vi "NewSolutionFitness.vi"(8 "error in (no error)":errorcluster, 10 "OSSP_Problem.lvclass":refnum<class "OSSP_Problem.lvclass">, 11 "GA in":refnum<class "GA.lvclass">) -> (0 "error out":errorcluster, 2 "OSSP_Problem out":refnum<class "OSSP_Problem.lvclass">, 3 "GA out":refnum<class "GA.lvclass">)   [LabVIEW 2013, in "GA.lvclass"]
uses:
  GA.lvclass
  OSSP_Problem.lvclass
  GA.lvclass/GA.ctl
  OSSP_Problem.lvclass/OSSP_Problem.ctl
  GanntChart_Class/Operation to Machine Job Tuple.vi
  GanntChart_Class/Check Other Machines for Schedule Time.vi
  GanntChart_Class/Schedule Job.vi
  GanntChart_Class/Find Gaps on Particular Machine.vi
  GanntChart_Class/Increment Number of Jobs on Machine.vi
  GanntChart_Class/Find Job On Other Machines.vi
  GanntChart.lvclass
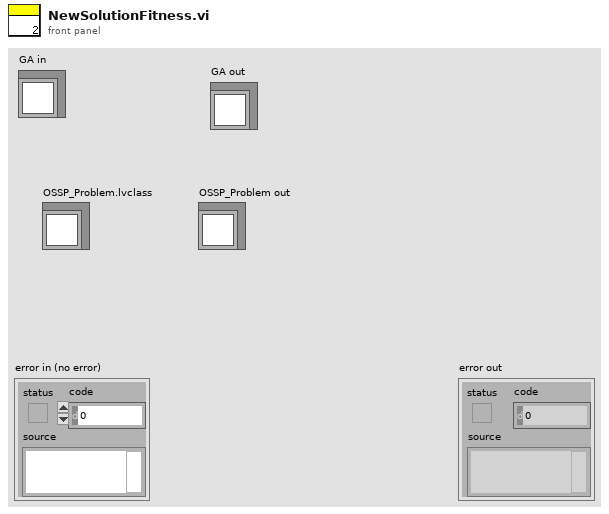
[diagram p1: front panel]
types:
  T1 = typedef "Solution_GA.ctl" = cluster{"Schedule":u16[], "Fitness":u16, "Fitness Valid?":bool}
  T2 = typedef "Scheduler Type.ctl" = enum16{"Non Delay Scheduler", "GT Active Scheduler", "My Scheduler"}
  T3 = typedef "Objective.ctl" = enum16{"Makespan", "Total Tardiness"}
  T4 = typedef "GanntChart_Element.ctl" = cluster{"Operation Number":i32, "Job Number":i32, "Start Time":i32, "Procesing Time":u16, "End Time":i32}
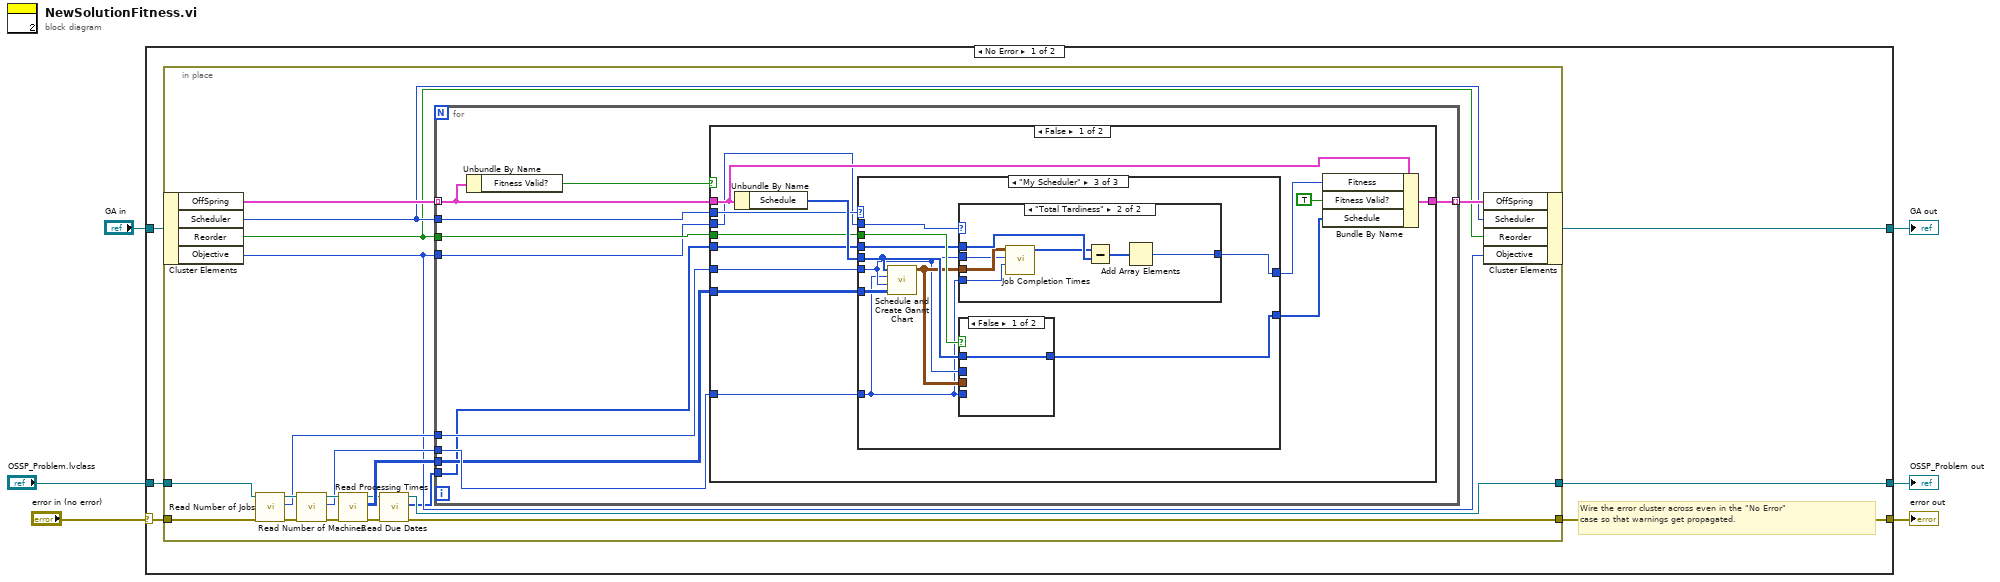
[diagram p0: block diagram]
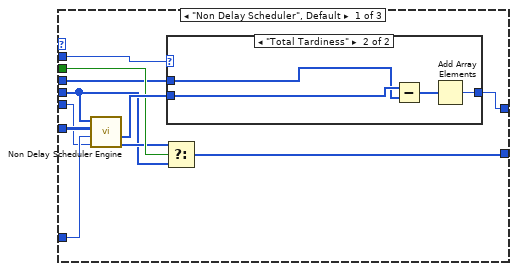
[diagram p2: hidden frame]
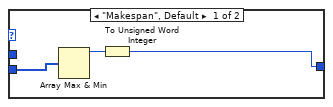
[diagram p3: hidden frame]
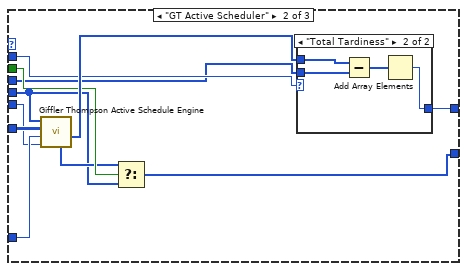
[diagram p4: hidden frame]
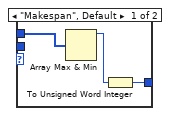
[diagram p5: hidden frame]
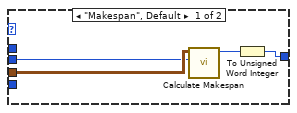
[diagram p6: hidden frame]
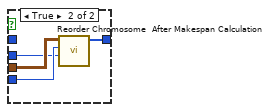
[diagram p7: hidden frame]
diagram:
  n1 = case shown="No Error" "error in (no error)" {
    selector: "error in (no error)" -> [w10 w120]
    tunnel: [w9 w120] -> w5
    tunnel: [w7 w119] -> w3
    tunnel: "GA in" -> [w8 w119]
    tunnel: "OSSP_Problem.lvclass" -> [w12 w118]
    tunnel: [w11 w118] -> w1
    frame No Error {
      # "Wire the error cluster across even in the \"No Error\"\ncase so that warnings get propagated."
      n2 = in-place {
        in-place-border: w12 -> [w31]
        in-place-border: [w16] -> w11
        in-place-border: w10 -> [w23]
        in-place-border: [w14] -> w9
        n3 = in-place-cluster #1(w8) -> ("OffSpring"=w21:T1[], "Scheduler"=w20:T2, "Reorder"=w19:bool, "Objective"=w18:T3)
        n4 = call-dynamic "Read Number of Jobs.vi"("error in (no error)"=w23, "OSSP_Problem in"=w31) -> ("error out"=w25:errorcluster, "Number of Jobs"=w28:i32, "OSSP_Problem out"=w30:refnum<class "OSSP_Problem.lvclass">)  [unwired: 7 in]
        n5 = call-dynamic "Read Number of Machines.vi"("error in (no error)"=w25, "OSSP_Problem in"=w30) -> ("error out"=w24:errorcluster, "Number of Machines"=w27:i32, "OSSP_Problem out"=w29:refnum<class "OSSP_Problem.lvclass">)  [unwired: 7 in]
        n6 = call-dynamic "Read Processing Times.vi"("error in (no error)"=w24, "OSSP_Problem in"=w29) -> ("error out"=w15:errorcluster, "Processing Times"=w26:u16[][], "OSSP_Problem out"=w17:refnum<class "OSSP_Problem.lvclass">)  [unwired: 7 in]
        n7 = call "Read Due Dates.vi"("error in (no error)"=w15, "OSSP_Problem in"=w17) -> ("error out"=w14:errorcluster, "Due Dates"=w13:u16[], "OSSP_Problem out"=w16:refnum<class "OSSP_Problem.lvclass">)  [unwired: 7 in]
        n8 = for {
          tunnel: w21 -> [w40] mode=indexing
          tunnel: [w39] -> w22 mode=indexing
          tunnel: w28 -> [w38]
          tunnel: w27 -> [w37]
          tunnel: w26 -> [w36]
          tunnel: w20 -> [w35]
          tunnel: w19 -> [w34]
          tunnel: w18 -> [w33]
          tunnel: w13 -> [w32]
          n9 = Unbundle By Name(w40) -> ("Fitness Valid?"=w41:bool)
          n10 = case shown="False" w41 {
            tunnel: w40 -> [w53 w117]
            tunnel: [w54 w117] -> w39
            tunnel: w38 -> [w48 _]
            tunnel: w37 -> [w50 _]
            tunnel: w36 -> [w51 _]
            tunnel: w35 -> [w46 _]
            tunnel: w34 -> [w44 _]
            tunnel: w33 -> [w43 _]
            tunnel: w32 -> [w42 _]
            frame False {
              n11 = Unbundle By Name(w53) -> ("Schedule"=w49:u16[])
              n12 = case shown="\"My Scheduler\"" w46 {
                tunnel: w51 -> [w65 w83 w100]
                tunnel: w50 -> [w64 w82 w91]
                tunnel: w49 -> [w57 w76 w97]
                tunnel: w48 -> [w63 w81 w95]
                tunnel: [w61 w79 w94] -> w47
                tunnel: [w58 w75 w99] -> w45
                tunnel: w44 -> [w60 w78 w98]
                tunnel: w43 -> [w56 w74 w93]
                tunnel: w42 -> [w55 w73 w92]
                frame "Non Delay Scheduler", Default {
                  n13 = call "Non Delay Scheduler Engine.vi"("Number of  Jobs"=w63, "Number of Machines"=w64, "Processing Times"=w65, "Schedule"=w57) -> ("Scheduled Jobs Order"=w59:u16[], "Job Completion Times"=w62:u16[])  [unwired: 3 in, 3 out]
                  n14 = Select(t=w59, s=w60, f=w57) -> (s? t:f=w58:u16[])
                  n15 = case shown="\"Total Tardiness\"" w56 {
                    tunnel: w62 -> [w68 w72]
                    tunnel: [w66 w69] -> w61
                    tunnel: w55 -> [_ w71]
                    frame "Makespan", Default {
                      n16 = Array Max & Min(array=w68) -> (max value=w67:u16)  [unwired: 3 out]
                      n17 = To Unsigned Word Integer(number=w67) -> (unsigned 16bit integer=w66:u16)
                    }
                    frame "Total Tardiness" {
                      n18 = Subtract(x=w72, y=w71) -> (x-y=w70:u16[])
                      n19 = Add Array Elements(numeric array=w70) -> (sum=w69:u16)
                    }
                  }
                }
                frame "GT Active Scheduler" {
                  n20 = call "Giffler Thompson Active Schedule Engine.vi"("Number of  Jobs"=w81, "Number of Machines"=w82, "Processing Times"=w83, "Schedule In"=w76) -> ("Job Completion Times"=w80:u16[], "Schedule Order"=w77:u16[])  [unwired: 3 in, 3 out]
                  n21 = Select(t=w77, s=w78, f=w76) -> (s? t:f=w75:u16[])
                  n22 = case shown="\"Total Tardiness\"" w74 {
                    tunnel: w80 -> [w86 w90]
                    tunnel: [w84 w87] -> w79
                    tunnel: w73 -> [_ w89]
                    frame "Makespan", Default {
                      n23 = Array Max & Min(array=w86) -> (max value=w85:u16)  [unwired: 3 out]
                      n24 = To Unsigned Word Integer(number=w85) -> (unsigned 16bit integer=w84:u16)
                    }
                    frame "Total Tardiness" {
                      n25 = Subtract(x=w90, y=w89) -> (x-y=w88:u16[])
                      n26 = Add Array Elements(numeric array=w88) -> (sum=w87:u16)
                    }
                  }
                }
                frame "My Scheduler" {
                  n27 = call "Schedule and Create Gannt Chart.vi"("Processing Times (Rows Mach.Cols Jobs)"=w100, "Number of Jobs"=w95, "Number of Machines"=w91, "Schedule"=w97) -> ("Gannt Chart Out"=w96:T4[][])  [unwired: 6 in, 1 out]
                  n28 = case shown="\"Total Tardiness\"" w93 {
                    tunnel: [w103 w110] -> w94
                    tunnel: w96 -> [w102 w108]
                    tunnel: w95 -> [w101 w107]
                    tunnel: w92 -> [_ w109]
                    tunnel: w91 -> [_ w106]
                    frame "Makespan", Default {
                      n29 = call "Calculate Makespan.vi"("Number of Jobs"=w101, "Gannt Chart In"=w102) -> ("Makespan"=w104:i32)  [unwired: 9 in]
                      n30 = To Unsigned Word Integer(number=w104) -> (unsigned 16bit integer=w103:u16)
                    }
                    frame "Total Tardiness" {
                      n31 = call "Job Completion Times.vi"("Number Of Machines"=w106, "Number Of Jobs"=w107, "Gannt Chart In"=w108) -> ("Job Completion Times"=w105:u16[])  [unwired: 8 in]
                      n32 = Subtract(x=w105, y=w109) -> (x-y=w111:u16[])
                      n33 = Add Array Elements(numeric array=w111) -> (sum=w110:u16)
                    }
                  }
                  n34 = case shown="False" w98 {
                    tunnel: [w112 w116] -> w99
                    tunnel: w96 -> [_ w115]
                    tunnel: w91 -> [_ w114]
                    tunnel: w95 -> [_ w113]
                    tunnel: w97 -> [w112 _]
                    frame False {
                    }
                    frame True {
                      n35 = call "Reorder Chromosome  After Makespan Calculation.vi"("Number Of  Jobs"=w113, "Number Of Machines"=w114, "Gannt Chart In"=w115) -> ("Reordered Chromosome"=w116:u16[])  [unwired: 8 in]
                    }
                  }
                }
              }
              n36 = Bundle By Name(cluster=w53, "Fitness"=w47, "Fitness Valid?"=TRUE, "Schedule"=w45) -> (w54:T1)
            }
            frame True {
            }
          }
        }
        n37 = in-place-cluster #1("OffSpring"=w22, "Scheduler"=w20, "Reorder"=w19, "Objective"=w18) -> (w7:refnum<class "GA.lvclass">)
      }
    }
    frame Error {
    }
  }
  "error out" <- w5
  "GA out" <- w3
  "OSSP_Problem out" <- w1
